vi "Inst.Krohn-Hite-7008.handleSetCommand.vi"(8 "error in (no error)":errorcluster, 9 "Data":variant, 10 "Command":string, 11 "Inst.Krohn-Hite-7008 in":refnum<class "Inst.Krohn-Hite-7008.lvclass">) -> (0 "error out":errorcluster, 3 "Inst.Krohn-Hite-7008 out":refnum<class "Inst.Krohn-Hite-7008.lvclass">)   [LabVIEW 2019, in "Inst.Krohn-Hite-7008.lvclass"]
uses:
  Inst.Krohn-Hite-7008.lvclass
  Inst.Krohn-Hite-7008.lvclass/Inst.Krohn-Hite-7008.ctl
  KH7008/typedefs/channelProperties--Cluster.ctl
  KH7008/typedefs/channel--enum.ctl
  KH7008/typedefs/gain--enum.ctl
  KH7008/typedefs/Input--Enum.ctl
  KH7008/typedefs/shunt--enum.ctl
  KH7008/typedefs/couple--Enum.ctl
  KH7008/typedefs/Filter--Enum.ctl
  Typedefs/setAllChannelsRequest--Cluster.ctl
  KH7008/typedefs/allChannelProperties--Array.ctl
  c4dadc50-be8b-432b-97b8-ac886381efa0.vi/1693475f-4e86-47ec-b72b-ebab137fdf19.vi
  c4dadc50-be8b-432b-97b8-ac886381efa0.vi/c53e0288-6dce-4a4b-a406-f7efad70ae81.vi
  <vilib>/Utility/Data Type/Get Type Information.vi
  <vilib>/JDP Science/JSONtext/JSON text to Variant.vi
  <vilib>/JDP Science/JSONtext/LVClass Serializer/JSONtext LVClass Serializer.lvclass
  KH7008/KH7008.lvlib
  <vilib>/JDP Science/JSONtext/JSONtext.lvlib
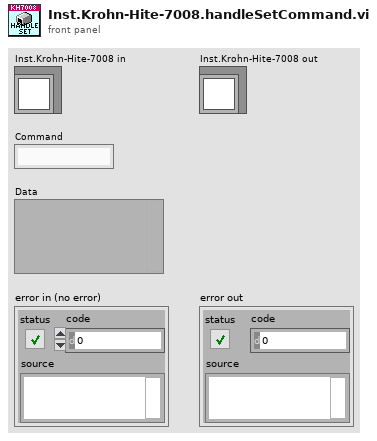
[diagram p1: front panel]
types:
  T1 = typedef "KH7008.lvlib/allChannelProperties--Array.ctl" = T2[]
  T2 = typedef "KH7008.lvlib/channelProperties--Cluster.ctl" = cluster{"channel":T3, "gain":T4, "input":T5, "shunt":T6, "couple":T7, "filter":T8}
  T3 = typedef "KH7008.lvlib/channel--enum.ctl" = enum16{"1", "2", "3", "4", "5", "6", "7", "8"}
  T4 = typedef "KH7008.lvlib/gain--enum.ctl" = enum16{"1x", "10x", "100x", "1000x"}
  T5 = typedef "KH7008.lvlib/input--enum.ctl" = enum16{"OFF", "SE+", "SE-", "DIFF"}
  T6 = typedef "KH7008.lvlib/shunt--enum.ctl" = enum16{"Open", "50", "500", "5k", "50k", "10M"}
  T7 = typedef "KH7008.lvlib/couple--enum.ctl" = enum16{"AC", "DC"}
  T8 = typedef "KH7008.lvlib/filter--enum.ctl" = enum16{"OFF", "ON"}
  T9 = typedef "Inst.Krohn-Hite-7008.lvclass/setAllChannelsRequest--Cluster.ctl" = cluster{"allChannelProperties":T1}
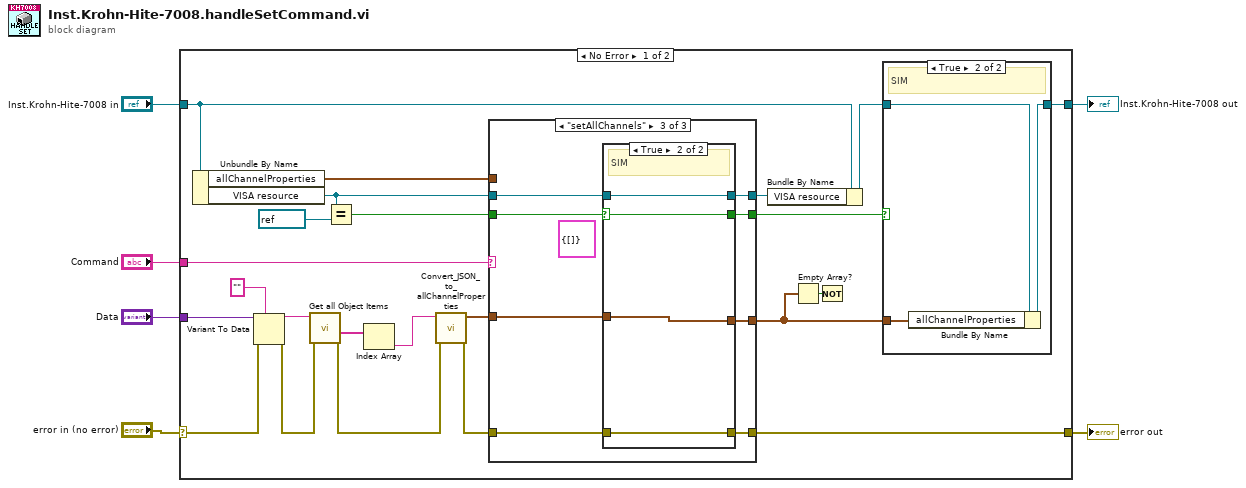
[diagram p0: block diagram]
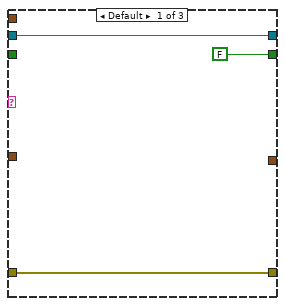
[diagram p2: hidden frame]
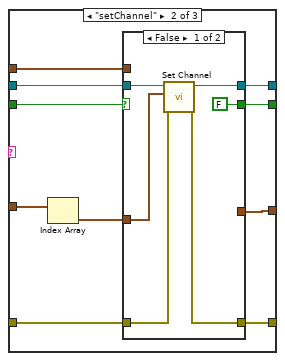
[diagram p3: hidden frame]
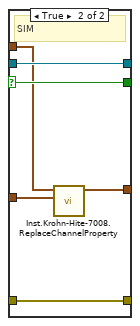
[diagram p4: hidden frame]
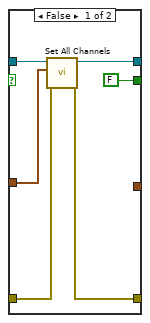
[diagram p5: hidden frame]
diagram:
  n1 = case shown="No Error" "error in (no error)" {
    selector: "error in (no error)" -> [w11 w77]
    tunnel: "Command" -> [w29 _]
    tunnel: "Data" -> [w13 _]
    tunnel: [w23 w78] -> w3
    tunnel: "Inst.Krohn-Hite-7008 in" -> [w28 w78]
    tunnel: [w27 w77] -> w1
    frame No Error {
      n2 = Unbundle By Name(w28) -> ("allChannelProperties"=w18:T1, "VISA resource"=w25:refnum<visa-resource-name>)
      n3 = Variant To Data(error in=w11, type="", Variant=w13) -> (data=w14:string, error out=w8:errorcluster)
      n4 = call <vilib>:"Get all Object Items.vi"("error in (no error)"=w8, "JSON"=w14) -> ("error out"=w9:errorcluster, "<JSON>"=w16:string[])  [unwired: 6 in, 2 out]
      n5 = Equal?(x=w25, y=refnum<visa-resource-name> "sim") -> (x = y?=w19:bool)
      n6 = Index Array(array=w16) -> (element=w15:string)  [unwired: 1 in]
      n7 = call "Convert_JSON_to_allChannelProperties.vi"("error in (no error)"=w9, "<JSON>"=w15) -> ("error out"=w10:errorcluster, "allChannelProperties"=w7:T1)  [unwired: 8 in]
      n8 = case shown="\"setAllChannels\"" w29 {
        tunnel: w10 -> [w31 w35 w56]
        tunnel: [w32 w42 w62] -> w24
        tunnel: [w31 w41 w61] -> w27
        tunnel: w25 -> [w32 w40 w60]
        tunnel: w19 -> [_ w39 w59]
        tunnel: [_ w36 w58] -> w20
        tunnel: [FALSE w38 w57] -> w17
        tunnel: w18 -> [_ w37 _]
        tunnel: w7 -> [_ w34 w55]
        frame Default {
        }
        frame "setChannel" {
          n9 = Index Array(array=w34) -> (element=w33:T2)  [unwired: 1 in]
          n10 = case shown="False" w39 {
            selector: w39 -> [_ w52]
            tunnel: w35 -> [w48 w53]
            tunnel: [w47 w54] -> w42
            tunnel: [w46 w53] -> w41
            tunnel: w40 -> [w45 w54]
            tunnel: w33 -> [w44 w51]
            tunnel: [FALSE w52] -> w38
            tunnel: w37 -> [_ w49]
            tunnel: [_ w50] -> w36
            frame False {
              n11 = call "Set Channel.vi"("error in (no error)"=w48, "channelParameter"=w44, "VISA Refnum in"=w45) -> ("error out"=w46:errorcluster, "VISA Refnum out"=w47:refnum<visa-resource-name>)  [unwired: 7 in]
            }
            frame True {
              # "SIM"
              n12 = call "Inst.Krohn-Hite-7008.ReplaceChannelProperty.vi"("channelProperties"=w51, "allChannelProperties"=w49) -> ("allChannelProperties"=w50:T1)  [unwired: 9 in]
            }
          }
        }
        frame "setAllChannels" {
          (unwired) T9 {"allChannelProperties"=[]} ("setAllChannelRequest")
          n13 = case shown="True" w59 {
            selector: w59 -> [_ w69]
            tunnel: w56 -> [w68 w71]
            tunnel: [w67 w72] -> w62
            tunnel: [w66 w71] -> w61
            tunnel: w60 -> [w65 w72]
            tunnel: w55 -> [w64 w70]
            tunnel: [_ w70] -> w58
            tunnel: [FALSE w69] -> w57
            frame False {
              n14 = call "Set All Channels.vi"("error in (no error)"=w68, "allChannelProperties"=w64, "VISA Refnum in"=w65) -> ("error out"=w66:errorcluster, "VISA Refnum out"=w67:refnum<visa-resource-name>)  [unwired: 6 in, 1 out]
            }
            frame True {
              # "SIM"
            }
          }
        }
      }
      n15 = Bundle By Name(cluster=w28, "VISA resource"=w24) -> (w22:refnum<class "Inst.Krohn-Hite-7008.lvclass">)
      n16 = Empty Array?(array=w20) -> (empty?=w21:bool)
      n17 = Not(x=w21) -> ()  [unwired: 1 out]
      n18 = case shown="True" w17 {
        tunnel: [w73 w76] -> w23
        tunnel: w22 -> [w73 w75]
        tunnel: w20 -> [_ w74]
        frame False {
        }
        frame True {
          # "SIM"
          n19 = Bundle By Name(cluster=w75, "allChannelProperties"=w74) -> (w76:refnum<class "Inst.Krohn-Hite-7008.lvclass">)
        }
      }
    }
    frame Error {
    }
  }
  "Inst.Krohn-Hite-7008 out" <- w3
  "error out" <- w1
